vi "Test_Copy_Array_To_Image_Greyscale.vi"(8 "error in (no error)":errorcluster, 11 "Test Case In":refnum<class "Image.lvclass">) -> (0 "error out":errorcluster, 3 "Test Case Out":refnum<class "Image.lvclass">)   [LabVIEW 2020, in "g_ar_toolkit.test.lvlib" / "Image.lvclass"]
uses:
  Image.lvclass
  Image.lvclass/Image.ctl
  g_ar_toolkit.image/g_ar_toolkit.image.lvlib
  g_ar_toolkit.image/CreateEmptyImageGreyscale.vi
  g_ar_toolkit.image/Image Size (Fixed).ctl
  4993e8ee-a06a-463a-9684-69129f64d5ce.vi
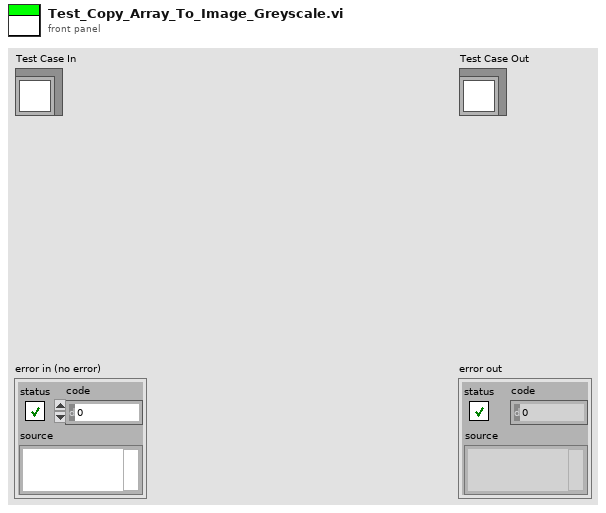
[diagram p1: front panel]
types:
  T1 = typedef "g_ar_toolkit.image.lvlib/Image Size (Fixed).ctl" = cluster{"Width":u16, "Height":u16}
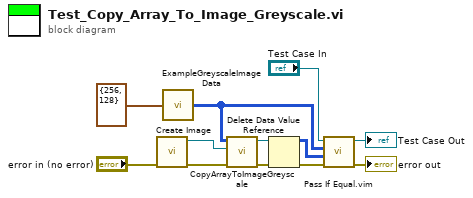
[diagram p0: block diagram]
diagram:
  n1 = call-poly "Create Image.vi"("error in (no error)"="error in (no error)") -> ("error out"=w4:errorcluster, "New Greyscale Image"=w3:refnum<data-value>)  [unwired: 9 in]
  n2 = call "ExampleGreyscaleImageData.vi"("Image Size"=T1 {"Width"=256, "Height"=128}) -> ("GreyscaleImage"=w1:u8[][])
  n3 = call "CopyArrayToImageGreyscale.vi"("error in (no error)"=w4, "Greyscale Destination Image"=w3, "Source"=w1) -> ("error out"=w7:errorcluster, "Greyscale Destination Image (duplicate)"=w2:refnum<data-value>)  [unwired: 7 in]
  n4 = Delete Data Value Reference(data value reference=w2, error in=w7) -> (data value=w9:u8[][], error out=w6:errorcluster)
  n5 = call "Pass If Equal.vim"("error in (no error)"=w6, "Actual"=w9, "Expected"=w1, "LUnit Test Case In"="Test Case In") -> ("error out"=→"error out":errorcluster, "LUnit Test Case Out"=→"Test Case Out":refnum<class "Image.lvclass">)  [unwired: 6 in]
